vi "getEventTask.vi"(8 "error in (no error)":errorcluster, 9 "pathOfSendEventSummaryState":path, 10 "pathLvLib":path, 11 "pathMonitor":path) -> (0 "error out":errorcluster)   [LabVIEW 2018]
doc: "Task of getting the event of LabVIEW. The event message is send by the CPP."
uses:
  SalProcess/SalProcess.lvclass
  LibReader/LibReader.lvclass
  SalProcess/SalProcess.lvclass/SalProcess.ctl
  CmpTool/checkData_priority.vi
  CmpTool/checkData_summaryState.vi
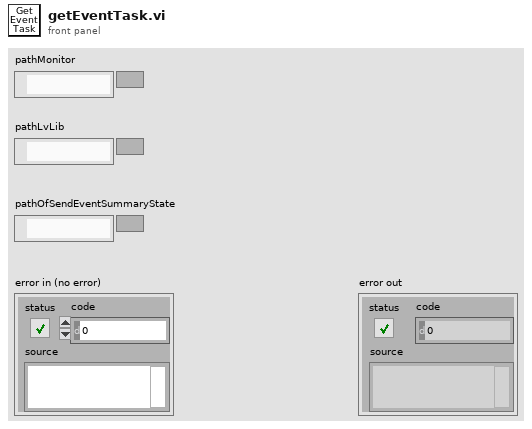
[diagram p1: front panel]
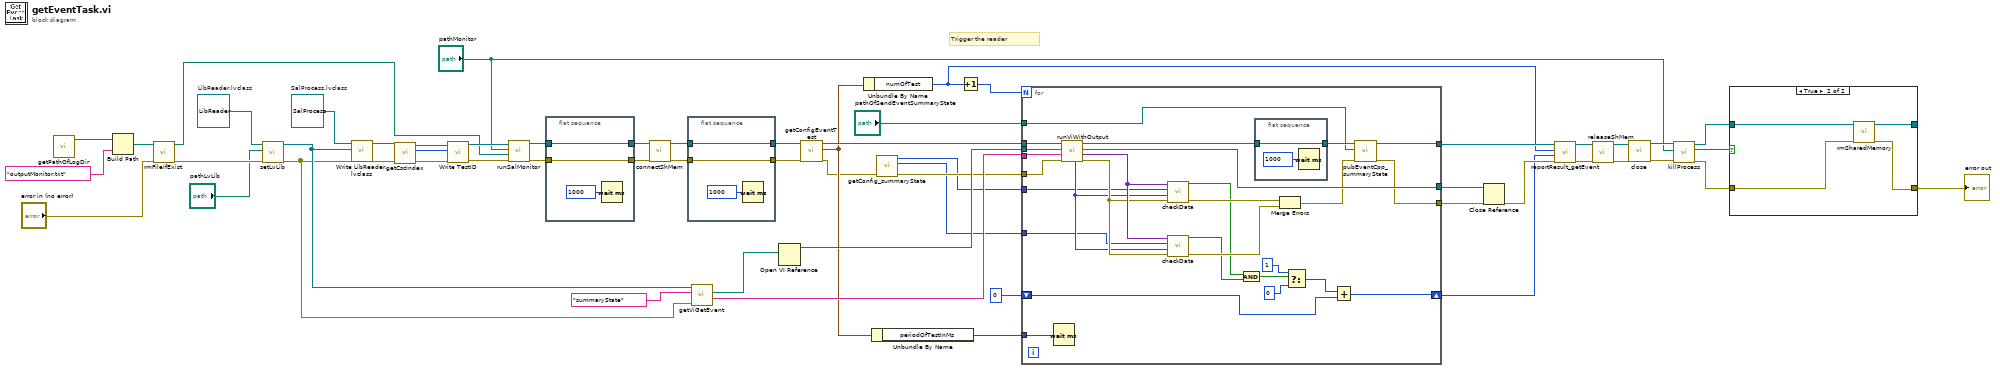
[diagram p0: block diagram]
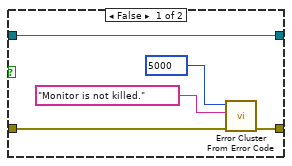
[diagram p2: hidden frame]
diagram:
  w44 = refnum<class "LibReader.lvclass"> refnum  # LibReader.lvclass
  w43 = refnum<class "SalProcess.lvclass"> refnum  # SalProcess.lvclass
  # "Trigger the reader"
  n1 = call "getPathOfLogDir.vi"() -> ("logDirPath"=w57:path)  [unwired: 11 in]
  n2 = Build Path(base path=w57, name or relative path="outputMonitor.txt") -> (appended path=w55:path)
  n3 = call "rmFileIfExist.vi"("error in (no error)"="error in (no error)", "path"=w55) -> ("error out"=w42:errorcluster, "pathDup"=w51:path)  [unwired: 8 in]
  n4 = call "setLvLib.vi"("error in (no error)"=w42, "pathLvLib"="pathLvLib", "LibReader in"=w44) -> ("error out"=w24:errorcluster, "LibReader out"=w26:refnum<class "LibReader.lvclass">)  [unwired: 7 in]
  n5 = call "Write LibReader.lvclass.vi"("error in (no error)"=w24, "LibReader.lvclass"=w26, "SalProcess in"=w43) -> ("error out"=w27:errorcluster, "SalProcess out"=w31:refnum<class "SalProcess.lvclass">)  [unwired: 7 in]
  n6 = call "getCscIndex.vi"("error in (no error)"=w27, "SalProcess in"=w31) -> ("error out"=w28:errorcluster, "cscIdx"=w29:i32, "SalProcess out"=w30:refnum<class "SalProcess.lvclass">)  [unwired: 7 in]
  n7 = call "Write TestID.vi"("error in (no error)"=w28, "TestID"=w29, "SalProcess in"=w30) -> ("error out"=w52:errorcluster, "SalProcess out"=w53:refnum<class "SalProcess.lvclass">)  [unwired: 7 in]
  n8 = call "runSalMonitor.vi"("error in (no error)"=w52, "pathOfOutput"=w51, "pathOfSalMonitor"="pathMonitor", "SalProcess in"=w53) -> ("error out"=w50:errorcluster, "SalProcess out"=w49:refnum<class "SalProcess.lvclass">)  [unwired: 6 in]
  n9 = flat-sequence {
    tunnel: w50 -> [w60]
    tunnel: w49 -> [w58]
    tunnel: [w60] -> w36
    tunnel: [w58] -> w37
    frame #0 {
      n10 = Wait (ms)(milliseconds to wait=u32 1000) -> ()  [unwired: 1 out]
    }
  }
  n11 = call "connectShMem.vi"("error in (no error)"=w36, "SalProcess in"=w37) -> ("error out"=w35:errorcluster, "SalProcess out"=w34:refnum<class "SalProcess.lvclass">)  [unwired: 7 in, 1 out]
  n12 = flat-sequence {
    tunnel: w35 -> [w62]
    tunnel: w34 -> [w63]
    tunnel: [w63] -> w17
    tunnel: [w62] -> w16
    frame #0 {
      n13 = Wait (ms)(milliseconds to wait=u32 1000) -> ()  [unwired: 1 out]
    }
  }
  n14 = call "getViGetEvent.vi"("error in (no error)"=w24, "name"="summaryState", "LibReader in"=w26) -> ("clusterNameOutput"=w19:string, "pathViGetEvent"=w23:path)  [unwired: 5 in, 2 out]
  n15 = Open VI Reference(vi path=w23) -> (vi reference=w22:refnum<vi>)  [unwired: 5 in, 1 out]
  n16 = call "getConfigEventTest.vi"("error in (no error)"=w16, "SalProcess in"=w17) -> ("error out"=w12:errorcluster, "configEventTest"=w14:cluster{"numOfTest":i32, "periodOfTestInMs":u32}, "SalProcess out"=w15:refnum<class "SalProcess.lvclass">)  [unwired: 7 in]
  n17 = Unbundle By Name(w14) -> ("numOfTest"=w1:i32)
  n18 = Unbundle By Name(w14) -> ("periodOfTestInMs"=w13:u32)
  n19 = call "getConfig_summaryState.vi"("error in (no error)"=w12) -> ("error out"=w11:errorcluster, "priority"=w9:i32, "summaryState"=w10:i32)  [unwired: 8 in]
  n20 = Increment(x=w1) -> (x+1=w2:i32)
  n21 = for {
    N: w2 -> [_]
    tunnel: w15 -> [w90]
    tunnel: [w69] -> w7
    tunnel: w11 -> [w88]
    tunnel: w22 -> [w89]
    tunnel: [w86] -> w21
    tunnel: [w67] -> w20
    tunnel: w19 -> [w87]
    tunnel: w10 -> [w82]
    tunnel: w9 -> [w81]
    shift-right: [w73] -> w3
    shift-left: 0 -> [w71]
    tunnel: w13 -> [w70]
    tunnel: "pathOfSendEventSummaryState" -> [w64]
    n22 = Wait (ms)(milliseconds to wait=w70) -> ()  [unwired: 1 out]
    n23 = call "runViWithOutput.vi"("error in (no error)"=w88, "clusterNameOutput"=w87, "referenceIn"=w89, "SalProcess in"=w90) -> ("error out"=w84:errorcluster, "variant"=w85:variant, "referenceOut"=w86:refnum<vi>, "SalProcess out"=w65:refnum<class "SalProcess.lvclass">, "function return"=w83:i32)  [unwired: 3 in]
    n24 = call-poly "checkData.vi"("error in (no error)"=w84, "function return"=w83, "valExpect"=w82, "variant"=w85) -> ("error out"=w80:errorcluster, "isExpected"=w78:bool)  [unwired: 6 in]
    n25 = call-poly "checkData.vi"("error in (no error)"=w84, "function return"=w83, "valExpect"=w81, "variant"=w85) -> ("error out"=w79:errorcluster, "isExpected"=w77:bool)  [unwired: 6 in]
    n26 = And(x=w78, y=w77) -> (x .and. y?=w76:bool)
    n27 = flat-sequence {
      tunnel: [w92] -> w66
      tunnel: w65 -> [w92]
      frame #0 {
        n28 = Wait (ms)(milliseconds to wait=u32 1000) -> ()  [unwired: 1 out]
      }
    }
    n29 = Merge Errors(w80, w79) -> (w68:errorcluster)
    n30 = Select(t=1, s=w76, f=0) -> (s? t:f=w72:i32)
    n31 = Add(x=w72, y=w71) -> (x+y=w73:i32)
    n32 = call "pubEventCpp_summaryState.vi"("error in (no error)"=w68, "pathOfSendEventSummaryState"=w64, "SalProcess in"=w66) -> ("error out"=w67:errorcluster, "SalProcess out"=w69:refnum<class "SalProcess.lvclass">)  [unwired: 7 in]
  }
  n33 = Close Reference(reference=w21, error in (no error)=w20) -> (error out=w4:errorcluster)
  n34 = call "reportResult_getEvent.vi"("error in (no error)"=w4, "timesSuccess"=w3, "timesTest"=w1, "SalProcess in"=w7) -> ("error out"=w5:errorcluster, "SalProcess out"=w6:refnum<class "SalProcess.lvclass">)  [unwired: 6 in]
  n35 = call "releaseShMem.vi"("error in (no error)"=w5, "SalProcess in"=w6) -> ("error out"=w32:errorcluster, "SalProcess out"=w33:refnum<class "SalProcess.lvclass">)  [unwired: 7 in, 1 out]
  n36 = call "close.vi"("error in (no error)"=w32, "SalProcess in"=w33) -> ("error out"=w40:errorcluster, "SalProcess out"=w41:refnum<class "SalProcess.lvclass">)  [unwired: 8 in]
  n37 = call "killProcess.vi"("error in (no error)"=w40, "pathOfProcess"="pathMonitor", "SalProcess in"=w41) -> ("error out"=w46:errorcluster, "isRemoved"=w48:bool, "SalProcess out"=w47:refnum<class "SalProcess.lvclass">)  [unwired: 6 in]
  n38 = case shown="True" w48 {
    tunnel: w47 -> [w97 w98]
    tunnel: w46 -> [w95 w99]
    tunnel: [w96 w101] -> w45
    tunnel: [w97 w100] -> _
    frame False {
      n39 = call <vilib>:"Error Cluster From Error Code.vi"("error in (no error)"=w95, "error message (\"\")"="Monitor is not killed." ("error message (\"\")"), "error code (0)"=5000) -> ("error out"=w96:errorcluster)  [unwired: 6 in]
    }
    frame True {
      n40 = call "rmSharedMemory.vi"("error in (no error)"=w99, "SalProcess in"=w98) -> ("error out"=w101:errorcluster, "SalProcess out"=w100:refnum<class "SalProcess.lvclass">)  [unwired: 7 in, 1 out]
    }
  }
  "error out" <- w45
